vi "XNET Read (Signal XY).vi"(0 "session in":refnum<k21>, 7 "number to read (-1)":i32=-1, 9 "time limit (none)":timestamp, 11 "error in (no error)":errorcluster) -> (4 "session out":refnum<k21>, 6 "data":T1(array[cluster]), 15 "error out":errorcluster)   [LabVIEW 2018]
doc: "Reads data from a session of Signal Input XY mode."
uses:
  nixlvapi.dll
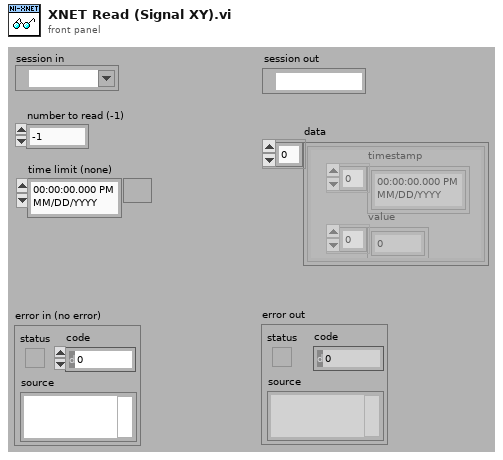
[diagram p1: front panel]
types:
  T1 = cluster{"timestamp":timestamp[], "value":dbl[]}[]
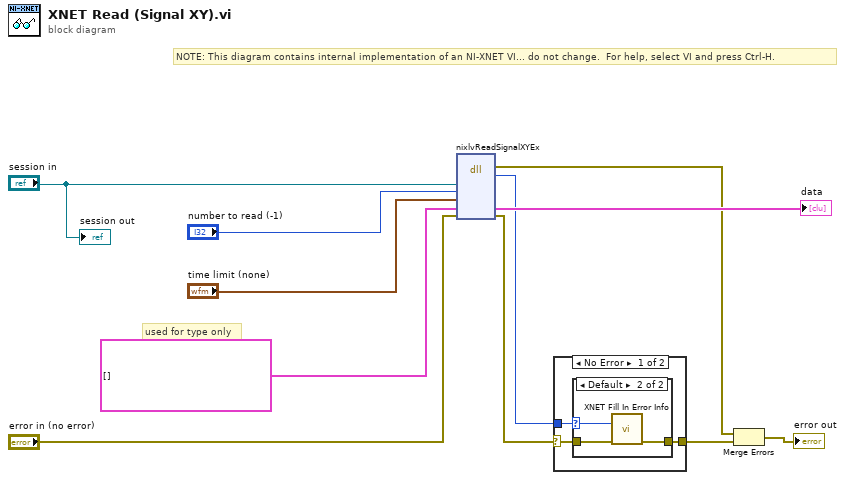
[diagram p0: block diagram]
diagram:
  # "used for type only"
  # "NOTE: This diagram contains internal implementation of an NI-XNET VI... do not change.  For help, select VI and press Ctrl-H."
  n1 = dll-call lib="nixlvapi.*" fn="nixlvReadSignalXYEx" label="Call Library"("sessionRef"="session in", "numberToRead"="number to read (-1)", "timeLimit"="time limit (none)", "lvData"=T1 [] ("data"), "errorInOut"="error in (no error)") -> (error out=w1:errorcluster, "return type"=w4:i32, "lvData"=→"data":T1, "errorInOut"=w3:errorcluster)  [unwired: 5 in, 2 out]
  n2 = case shown="No Error" w3 {
    selector: w3 -> [w12 w19]
    tunnel: [w14 w19] -> w11
    tunnel: w4 -> [w13 _]
    frame No Error {
      n3 = case shown="Default" w13 {
        selector: w13 -> [_ w16]
        tunnel: w12 -> [w15 w17]
        tunnel: [w15 w18] -> w14
        frame 0 {
        }
        frame Default {
          n4 = call "XNET Fill In Error Info.vi"("status code"=w16, "error in"=w17) -> ("error out"=w18:errorcluster)  [unwired: 13 out]
        }
      }
    }
    frame Error {
    }
  }
  n5 = Merge Errors(w1, w11) -> (→"error out":errorcluster)
  "session out" <- "session in"
